vi "GetNumFromName.vi"(8 "error in (no error)":errorcluster, 10 "name":string, 11 "dvotAFTKinetics":refnum<class "dvotAFTKinetics.lvclass">) -> (0 "error out":errorcluster, 2 "Numeric":i32, 3 "dvotAFTKinetics":refnum<class "dvotAFTKinetics.lvclass">)   [LabVIEW 2012, in "dvotAFTKinetics.lvclass"]
uses:
  dvotAFTKinetics.lvclass
  Constants/dvotAFTConstants.vi
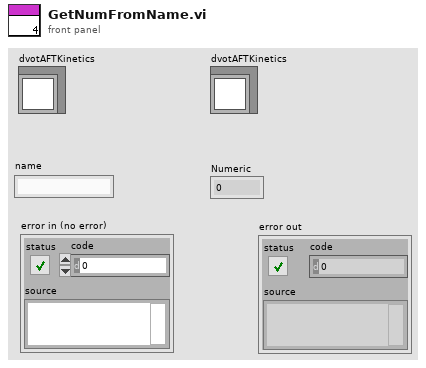
[diagram p1: front panel]
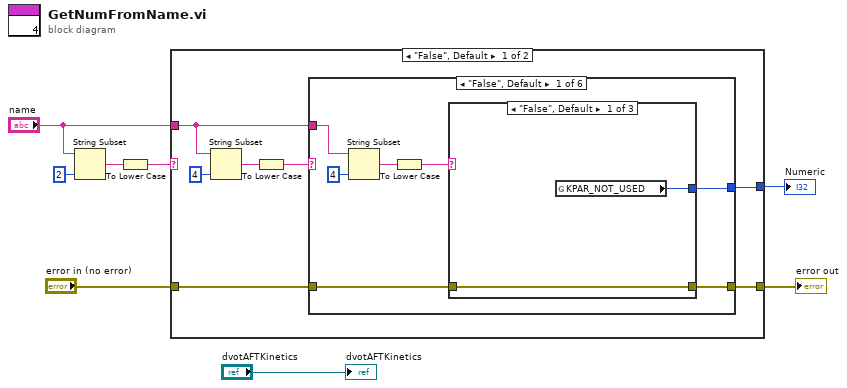
[diagram p0: block diagram]
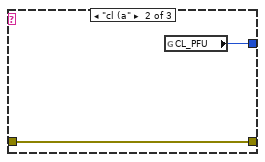
[diagram p2: hidden frame]
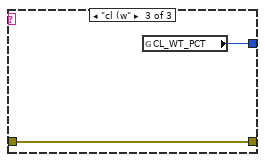
[diagram p3: hidden frame]
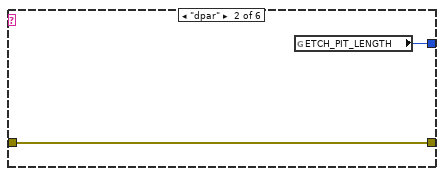
[diagram p4: hidden frame]
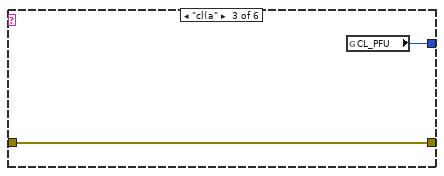
[diagram p5: hidden frame]
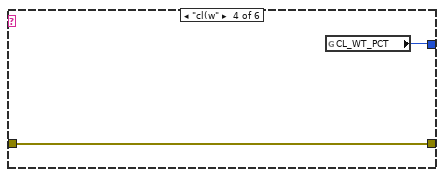
[diagram p6: hidden frame]
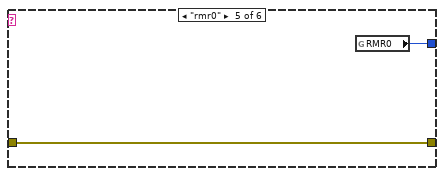
[diagram p7: hidden frame]
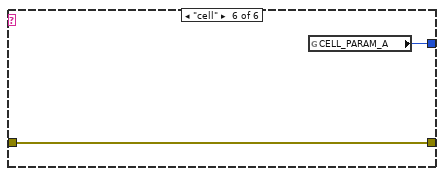
[diagram p8: hidden frame]
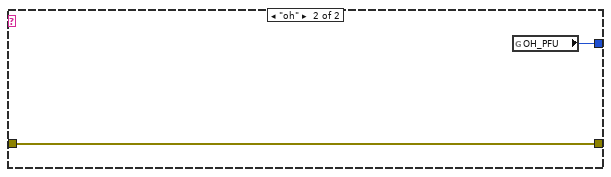
[diagram p9: hidden frame]
diagram:
  n1 = String Subset(string="name", length (rest)=2 ("length (rest)")) -> (substring=w8:string)  [unwired: 1 in]
  n2 = To Lower Case(string=w8) -> (all lower case string=w6:string)
  n3 = case shown="\"False\", Default" w6 {
    tunnel: "name" -> [w11 _]
    tunnel: [w12 w40] -> w4
    tunnel: "error in (no error)" -> [w10 w39]
    tunnel: [w9 w39] -> w1
    frame "False", Default {
      n4 = String Subset(string=w11, length (rest)=4 ("length (rest)")) -> (substring=w15:string)  [unwired: 1 in]
      n5 = To Lower Case(string=w15) -> (all lower case string=w13:string)
      n6 = case shown="\"False\", Default" w13 {
        tunnel: [w22 w30 w32 w34 w36 w38] -> w12
        tunnel: w11 -> [w19 _ _ _ _ _]
        tunnel: w10 -> [w17 w29 w31 w33 w35 w37]
        tunnel: [w16 w29 w31 w33 w35 w37] -> w9
        frame "False", Default {
          n7 = String Subset(string=w19, length (rest)=4 ("length (rest)")) -> (substring=w21:string)  [unwired: 1 in]
          n8 = To Lower Case(string=w21) -> (all lower case string=w18:string)
          n9 = case shown="\"False\", Default" w18 {
            tunnel: [w24 w26 w28] -> w22
            tunnel: w17 -> [w23 w25 w27]
            tunnel: [w23 w25 w27] -> w16
            frame "False", Default {
              n10 = global read "dvotAFTConstants.vi" "KPAR_NOT_USED"() -> (w24:i32)
            }
            frame "cl (a" {
              n11 = global read "dvotAFTConstants.vi" "CL_PFU"() -> (w26:i32)
            }
            frame "cl (w" {
              n12 = global read "dvotAFTConstants.vi" "CL_WT_PCT"() -> (w28:i32)
            }
          }
        }
        frame "dpar" {
          n13 = global read "dvotAFTConstants.vi" "ETCH_PIT_LENGTH"() -> (w30:i32)
        }
        frame "cl(a" {
          n14 = global read "dvotAFTConstants.vi" "CL_PFU"() -> (w32:i32)
        }
        frame "cl(w" {
          n15 = global read "dvotAFTConstants.vi" "CL_WT_PCT"() -> (w34:i32)
        }
        frame "rmr0" {
          n16 = global read "dvotAFTConstants.vi" "RMR0"() -> (w36:i32)
        }
        frame "cell" {
          n17 = global read "dvotAFTConstants.vi" "CELL_PARAM_A"() -> (w38:i32)
        }
      }
    }
    frame "oh" {
      n18 = global read "dvotAFTConstants.vi" "OH_PFU"() -> (w40:i32)
    }
  }
  "Numeric" <- w4
  "error out" <- w1
  "dvotAFTKinetics" <- "dvotAFTKinetics"
